vi "command to string.vi"(11 "commands":T1) -> (3 "command string":string)   [LabVIEW 2013, in "module execution process.lvlib"]
uses:
  module execution process.lvlib
  command commands to rtexe process.ctl
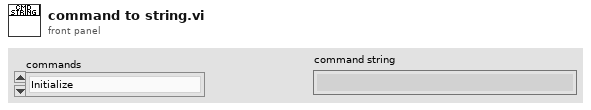
[diagram p1: front panel]
types:
  T1 = typedef "module execution process.lvlib/command commands to rtexe process.ctl" = enum16{"Initialize", "Add Search Paths", "Load from File", "Unload File", "Open All Engines", "Open Single Engine", "Initialize All Engines", "Initialize Single Engine", "Start All", "Start Single", "Pause All", "Pause Single", "Stop All", "Stop Single", "Close All", "Close Single", "Set Safe State All", "Set Safe State Single", "Get Status", "Exit", "Error", "Load Bitfile", "Unload Bitfile", "Clear Faults Single", "Clear Faults All"}
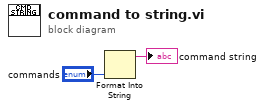
[diagram p0: block diagram]
diagram:
  n1 = Format Into String("commands") -> (resulting string=→"command string":string)  [unwired: 3 in, 1 out]
